vi "N-Channel N-Samples (2D DBL).vi"() -> ()   [LabVIEW 2019]
uses:
  <vilib>/DAQmx/read.llb/DAQmx Read (Analog 2D DBL NChan NSamp).vi
  <vilib>/DAQmx/create/channels.llb/DAQmx Create Channel (AI-Voltage-Basic).vi
  <vilib>/DAQmx/configure/timing.llb/DAQmx Timing (Sample Clock).vi
  <vilib>/DAQmx/miscellaneous.llb/DAQmx Fill In Error Info.vi
  <resource>/objmgr/daqmx.rc
panel:
  out "2D Array Indicator":dbl[][](array[numeric])
  out "Waveform Chart":dbl[][](graph)=[[2.0496230964079714, 1.4590899380474258, 1.1688589129306926], [1.792809839167455, 1.6428113650929288, 1.063875240333262], [1.977294228949858, 1.4178899502548294, 1.2041077913754692], [1.772057252723777, 1.6145817438276315, 1.1557359538560137], [1.804254280220954, 1.4838099307229835, 1.2335581530198065], [1.9325846125675221, 1.425977355265969, 0.957060457167272], [1.8865016632587663, 1.5289773247474594, 1.2024292733542894], [2.006744590594195, 1.5054780724509416, 1.108890041810358], [2.000793481246376, 1.3791314432203132, 0.9949034089175085], [1.7641224402600177, 1.5585802789391765, 1.010773033845027], [1.9341105380413222, 1.6245002594073306, 1.0701315347758416], [1.8980986968596454, 1.5283669545579395, 0.9697256385998108], [1.8352305673390912, 1.3620410779137546, 1.1365092928861353], [1.987670522171697, 1.4418469801934874, 1.0683004242072818], [1.9989623706778161, 1.5900143436994538, 0.934324167607654], [1.8655964842677084, 1.4720603045747245, 1.0792870876186407], [1.9122898037659841, 1.4857936338389233, 1.1467329935605945], [1.7418439283425398, 1.3936277352214117, 1.1227759636219368], [1.814020203253273, 1.4423047578356274, 1.1482589190343944], [1.8874172185430464, 1.4397106845301675, 1.1658070619830927], [1.8831446272164067, 1.3383892330698568, 1.08600115970336], [1.8190557573168127, 1.368144779808954, 1.0686056093020417], [1.9718008972441785, 1.424298837244789, 1.0715048677022614], [1.9710379345072786, 1.598406933805353, 0.9096041749320963], [1.7139194921720022, 1.4496292001098667, 0.9318826868495743], [1.9399090548417615, 1.5921506393627736, 1.0080263679921873], [1.7699209570604573, 1.381420331431013, 0.9009063997314372], [1.8753624073000275, 1.4758751182592242, 0.9627063814203314], [1.8892483291116062, 1.5924558244575335, 1.1323892941068758], [1.9069490646076845, 1.4687032685323649, 1.0504470961638233], [1.8732261116367077, 1.2892544328135014, 0.9527878658406324], [1.8730735190893277, 1.5356913968321788, 1.0397656178472243], [1.902829065828425, 1.5253151036103396, 0.945158238471633], [1.8997772148808252, 1.3528855250709555, 0.8984649189733573], [1.9202246162297434, 1.3434247871333964, 1.0531937620166631], [1.695913571581164, 1.5047151097140417, 1.1447492904446548], [1.9379253517258217, 1.4616840113528855, 0.8897671437726982], [1.8291268654438917, 1.4529862361522263, 1.1578722495193334], [1.9544053468428602, 1.381878109073153, 1.0357982116153448], [1.8515579699087497, 1.4844203009125034, 1.0507522812585832], [1.6920987578966644, 1.509292886135441, 1.0930204168828395], [1.9147312845240638, 1.2579729606006043, 0.9648426770836512], [1.705374309518723, 1.3516647846919156, 1.1029389324625385], [1.7534409619434186, 1.52302621539964, 1.096987823114719], [1.84789574877163, 1.2689596240119632, 0.9541611987670522], [1.7032380138554033, 1.2480544450209052, 1.0696737571337016], [1.7998290963469343, 1.3875240333262124, 0.9515671254615925], [1.8552201910458692, 1.4752647480697043, 0.9192175054170354], [1.8445387127292703, 1.5352336191900389, 0.9071626941740165], [1.7909787285988952, 1.2878810998870815, 0.968047120578631], [1.8315683462019714, 1.4183477278969696, 0.9179967650379955], [1.8291268654438917, 1.3315225684377574, 0.9793389690847499], [1.8506424146244698, 1.4864040040284432, 0.9111301004058961], [1.8674275948362682, 1.358073671681875, 1.0202337717825862], [1.7647328104495377, 1.2656025879696036, 1.044648579363384], [1.6786706137272256, 1.4389477217932676, 0.8099612414929654], [1.695150608844264, 1.4079714346751304, 0.9442426831873532], [1.7459639271217993, 1.426129947813349, 0.8490249336222419], [1.903134250923185, 1.4503921628467666, 1.0206915494247262], [1.728263191625721, 1.2985625782036805, 0.9382915738395337], [1.6559343241676077, 1.337626270332957, 0.8296456801049836], [1.6965239417706839, 1.3119907223731193, 1.0574663533433026], [1.6003906369212928, 1.4745017853328044, 0.8018738364818262], [1.7770928067873164, 1.4621417889950254, 0.9065523239844966], [1.760917996765038, 1.4735862300485245, 1.073946348460341], [1.8454542680135502, 1.249580370494705, 1.0556352427747429], [1.8408764915921507, 1.1912900173955503, 0.9602649006622517], [1.6621906186101871, 1.2094485305337688, 0.9547715689565721], [1.8057802056947538, 1.337015900143437, 0.8429212317270425], [1.7589342936490981, 1.2982573931089205, 0.9389019440290536], [1.6678365428632465, 1.4319284646137882, 0.7687612537003693], [1.717429120761742, 1.3324381237220375, 0.97872859889523], [1.7383342997528, 1.4278084658345287, 0.7548753318887905], [1.7766350291451765, 1.207464827417829, 0.8069093905453658], [1.6893520920438245, 1.401715140232551, 0.8729819635608996], [1.7703787347025972, 1.4052247688222907, 1.031983397930845], [1.6158024842066714, 1.3667714468825343, 0.9190649128696554], [1.8079165013580736, 1.2868129520554217, 0.9646900845362713], [1.6374706259346294, 1.314279610583819, 0.7527390362254708], [1.6692098757896665, 1.1691640980254525, 0.8868678853724784], [1.6875209814752647, 1.261787774285104, 0.9971922971282082], [1.5604113895077365, 1.3863032929471724, 0.8954130680257576], [1.6109195226905118, 1.1764885402996919, 0.8285775322733238], [1.6774498733481857, 1.4075136570329905, 0.8178960539567247], [1.8033387249366741, 1.1914426099429303, 0.8165227210303049], [1.8124942777794733, 1.2384411145359662, 0.7480086672566911], [1.7775505844294566, 1.1926633503219704, 0.913724173711356], [1.5301980651264993, 1.3428144169438765, 0.825830866420484], [1.6054261909848322, 1.3451033051545762, 0.8124027222510453], [1.6991180150761436, 1.3650929288613545, 0.826288644062624], [1.7670216986602374, 1.3003936887722403, 0.9662160100100711], [1.5895565660573137, 1.131168553727836, 0.7670827356791894], [1.6031373027741325, 1.3098544267097996, 0.8284249397259438], [1.5240943632312998, 1.2036500137333292, 0.7240516373180333], [1.7290261543626209, 1.1070589312417982, 0.9436323129978332], [1.5916928617206336, 1.3824884792626728, 0.7036042359691153], [1.7848750267036957, 1.346629230628376, 0.7521286660359509], [1.563921018097476, 1.1549729911191138, 0.7942442091128269], [1.7876216925565356, 1.3399151585436568, 0.9152500991851558], [1.6267891476180303, 1.08600115970336, 0.9396649067659536], [1.771446882534257, 1.1441389202551346, 0.9147923215430158], [1.5825373088778345, 1.3055818353831599, 0.6946012756736961], [1.5686513870662557, 1.1772515030365918, 0.9314249092074343], [1.73970763267922, 1.1685537278359326, 0.7600634784997101], [1.5619373149815363, 1.292764061403241, 0.9329508346812342], [1.717581713309122, 1.128269295327616, 0.6982634968108158], [1.6278572954496902, 1.2744529557176427, 0.9063997314371166], [1.4951017792291024, 1.2630085146641439, 0.7371745963927122], [1.4766380809961241, 1.1674855800042725, 0.9208960234382153], [1.6582232123783074, 1.3133640552995391, 0.8124027222510453], [1.5594958342234566, 1.152378917813654, 0.9169286172063357], [1.5952024903103732, 1.1154515213476974, 0.7209997863704337], [1.5506454664754172, 1.163060396130253, 0.749687185277871], [1.4766380809961241, 1.2344737083040864, 0.6935331278420362], [1.7117831965086825, 1.0626544999542222, 0.6682027649769585], [1.6933194982757043, 1.1105685598315378, 0.7773064363536485], [1.6782128360850856, 1.1680959501937926, 0.684377574999237], [1.6319772942289499, 1.3016144291512803, 0.8011108737449263], [1.4885402996917632, 1.19602038636433, 0.6324961088900418], [1.5906247138889738, 1.0403759880367442, 0.7918027283547472], [1.5659047212134158, 1.1232337412640767, 0.8751182592242195], [1.609698782311472, 1.3037507248146, 0.880458998382519], [1.4645832697531052, 1.1482589190343944, 0.6122013000885037], [1.4598529007843257, 1.1975463118381298, 0.6041138950773645], [1.4923551133762627, 1.250648518326365, 0.6295968504898221], [1.6133610034485917, 1.2971892452772606, 0.7138279366435744], [1.6928617206335643, 1.2111270485549486, 0.6306649983214819], [1.6844691305276651, 1.0197759941404463, 0.8867152928250984], [1.4323862422559281, 1.19647816400647, 0.6486709189123203], [1.674245429853206, 1.237830744346446, 0.7324442274239327], [1.63167210913419, 1.2022766808069094, 0.804620502334666], [1.555070650349437, 1.163212988677633, 0.6375316629535813], [1.6452528458510087, 1.077150791955321, 0.7486190374462112], [1.3948484756004518, 1.1152989288003174, 0.8285775322733238], [1.5710928678243354, 1.1009552293465987, 0.6002990813928648], [1.6130558183538315, 1.2340159306619465, 0.7968382824182867], [1.6823328348643452, 1.2707907345805232, 0.7515182958464308], [1.5901669362468338, 1.0889004181035797, 0.6591998046815394], [1.3846247749259926, 1.0037537766655475, 0.7267983031708731], [1.3823358867152928, 1.1554307687612537, 0.5595568712424085], [1.5150914029358806, 1.2424085207678457, 0.6707968382824183], [1.444898831141087, 0.9802545243690298, 0.6814783165990173], [1.5852839747306742, 1.0681478316599018, 0.5703909421063875], [1.4801477095858637, 1.098666341135899, 0.6944486831263161], [1.4398632770775475, 1.1455122531815547, 0.6692709128086184], [1.4505447553941466, 1.0248115482039857, 0.6099124118778039], [1.6159550767540514, 1.0567033906064027, 0.7219153416547136], [1.5465254676961577, 1.0557878353221228, 0.7379375591296121], [1.4592425305948058, 1.0895107882930997, 0.8192693868831447], [1.5381328775902585, 1.1360515152439954, 0.5378887295144505], [1.5478988006225776, 1.0504470961638233, 0.8011108737449263], [1.4841151158177435, 0.9833063753166296, 0.7771538438062685], [1.5939817499313333, 1.2140263069551682, 0.5423139133884701], [1.3719595934934539, 1.1838129825739312, 0.5117954039124729], [1.5205847346415602, 1.1449018829920348, 0.630512405774102], [1.349070711386456, 1.0928678243354595, 0.6881923886837367], [1.4313180944242683, 1.0611285744804224, 0.7553331095309305], [1.5225684377575, 1.043427838984344, 0.500198370311594], [1.4973906674398023, 1.0951567125461592, 0.6622516556291391], [1.381878109073153, 1.119113742484817, 0.6460768456068605], [1.5578173162022766, 1.0846278267769403, 0.5041657765434736], [1.3794366283150732, 1.1143833735160376, 0.7475508896145512], [1.3655507065034944, 1.0255745109408856, 0.7116916409802545], [1.4217047639393292, 1.1421552171391949, 0.5710013122959074], [1.5846736045411542, 1.1893063142796105, 0.7097079378643147], [1.5250099185155797, 1.1647389141514328, 0.5536057618945891], [1.5613269447920164, 1.1700796533097324, 0.6990264595477157], [1.4914395580919828, 0.9918515579699088, 0.5252235480819116], [1.3156529435102389, 0.9384441663869136, 0.5066072573015534], [1.3306070131534775, 0.9042634357737968, 0.5694753868221076], [1.545152134769738, 1.1581774346140934, 0.6540116580706198], [1.2970366527298807, 1.1140781884212776, 0.630054628131962], [1.5623950926236763, 1.1221655934324168, 0.6021301919614246], [1.293374431592761, 1.0362559892574847, 0.6495864741966002], [1.4065981017487106, 1.012451551866207, 0.685750907925657], [1.3306070131534775, 1.0245063631092257, 0.7147434919278542], [1.5582750938444165, 1.1256752220221564, 0.6324961088900418], [1.477553636280404, 0.9967345194860683, 0.4518265327921384], [1.5268410290841394, 1.0731833857234412, 0.5714590899380474], [1.5166173284096804, 0.9300515762810144, 0.6648457289345988], [1.476943266090884, 1.0890530106509597, 0.44724875637073885], [1.3771477401043732, 1.1278115176854762, 0.5259865108188116], [1.3773003326517532, 0.9155552842799157, 0.5667287209692679], [1.294595171971801, 0.8458204901272622, 0.48509170812097535], [1.30481887264626, 0.8986175115207373, 0.6961272011474959], [1.2649922177800836, 0.9936826685384685, 0.5796990874965666], [1.381572923978393, 1.076235236671041, 0.6897183141575366], [1.2765892513809625, 0.9843745231482894, 0.4426709799493393], [1.2753685110019226, 1.1014130069887387, 0.6497390667439802], [1.3441877498702963, 0.9897152623065889, 0.46571245460371713], [1.4200262459181494, 1.0521256141850033, 0.6849879451887569], [1.3704336680196538, 1.0472426526688436, 0.6064027832880642], [1.41285439619129, 1.0818811609241004, 0.631275368511002], [1.466872157963805, 1.0469374675740837, 0.576647236548967], [1.403698843348491, 0.9912411877803888, 0.6170842616046632], [1.5111239967040009, 0.9952085940122685, 0.44709616382335887], [1.4937284463026825, 1.0930204168828395, 0.38529618213446454], [1.336710715048677, 0.8883938108462782, 0.5926694540238655], [1.3969847712637715, 0.8359019745475631, 0.3985717337565233], [1.3884395886104923, 0.9266945402386547, 0.5159154026917325], [1.3753166295358135, 1.0812707907345804, 0.4664754173406171], [1.260414441358684, 1.0364085818048647, 0.4686117130039369], [1.317178868984039, 1.0400708029419843, 0.6051820429090243], [1.41315958128605, 0.8420056764427626, 0.564287240211188], [1.1970885341959898, 0.7966856898709067, 0.37003692739646593], [1.2634662923062838, 0.9276100955229346, 0.5041657765434736], [1.2866603595080417, 1.0203863643299662, 0.48295541245765555], [1.3121433149204993, 0.9207434308908353, 0.6234931485946227], [1.4056825464644307, 1.0289315469832454, 0.4881435590685751], [1.337168492690817, 0.8362071596423231, 0.4858546708578753], [1.1700796533097324, 0.9607226783043916, 0.5957213049714651], [1.292306283761101, 0.9918515579699088, 0.6070131534775841], [1.2088381603442488, 0.858790856654561, 0.41657765434736166], [1.2298959318826868, 0.9595019379253518, 0.4425183874019593], [1.2706381420331432, 1.0350352488784447, 0.6231879634998627], [1.2651448103274636, 1.0234382152775658, 0.45365764336069825], [1.4096499526963102, 0.967284157841731, 0.39063692129276406], [1.3518173772392956, 0.7689138462477493, 0.6031983397930845], [1.2158574175237282, 0.9617908261360515, 0.3553880428479873], [1.2709433271279031, 1.0112308114871669, 0.575579088717307], [1.2259285256508072, 0.9912411877803888, 0.4791405987731559], [1.4050721762749108, 0.9804071169164098, 0.402233954893643], [1.4101077303384502, 0.8595538193914609, 0.39216284676656393], [1.2952055421613209, 0.8928189947202979, 0.42649616992706074], [1.3455610827967162, 0.9686574907681509, 0.4142887661366619], [1.3084810937833795, 0.7454145939512314, 0.41596728415784173], [1.3824884792626728, 0.9152500991851558, 0.3979613635670034], [1.2166203802606281, 0.9669789727469711, 0.3573717459639271], [1.3234351634266182, 0.8606219672231208, 0.38453321939756463], [1.3280129398480178, 0.8169804986724448, 0.4770043031098361], [1.208227790154729, 0.8346812341685232, 0.41596728415784173], [1.1767937253944518, 0.7452620014038515, 0.3741569261757256], [1.1713003936887723, 0.6944486831263161, 0.2708517715994751], [1.184881130405591, 0.7940916165654469, 0.554826502273629], [1.2298959318826868, 0.7867671742912076, 0.3944517349772637], [1.313974425489059, 0.9143345439008759, 0.36255989257484666], [1.2445448164311654, 0.7155064546647542, 0.3514206366161077], [1.349375896481216, 0.8970915860469375, 0.34180730613116855], [1.1606189153721733, 0.9112826929532761, 0.42847987304300056], [1.1500900296029541, 0.9372234260078738, 0.49684133426923427], [1.2787255470442824, 0.7902768028809473, 0.3563035981322672], [1.1934263130588703, 0.8766441846980193, 0.5380413220618305], [1.292916653950621, 0.8027893917661062, 0.47029023102511675], [1.1720633564256722, 0.8717612231818598, 0.3979613635670034], [1.0794396801660207, 0.8507034516434218, 0.4971465193639943], [1.1116367076631977, 0.8107242042298655, 0.2739036225470748], [1.1935789056062502, 0.836817529831843, 0.511490218817713], [1.1981566820276497, 0.8339182714316232, 0.25513473921933655], [1.317178868984039, 0.7197790459913938, 0.45152134769737845], [1.1799981688894314, 0.8919034394360179, 0.260628070925016], [1.3135166478469191, 0.7560960722678305, 0.2897732474745933], [1.0701315347758416, 0.684377574999237, 0.37888729514450514], [1.2320322275460067, 0.8098086489455855, 0.23133030182805872], [1.066774498733482, 0.7571642200994904, 0.4112369151890622], [1.0885952330088198, 0.6787316507461776, 0.42344431897946105], [1.2611774040955839, 0.8665730765709403, 0.2996917630542924]]
  out "Waveform Graph":dbl[][](graph)
  out "Actual Sample Rate (Hz)":dbl
  in  "Desired Sample Rate (Hz)":dbl=2560.0
  in  "Number of Samples":i32=256
  in  "Stop":bool
  in  "Physical Channels":tag="PCI-6221/ai0, PCI-6221/ai2:3"
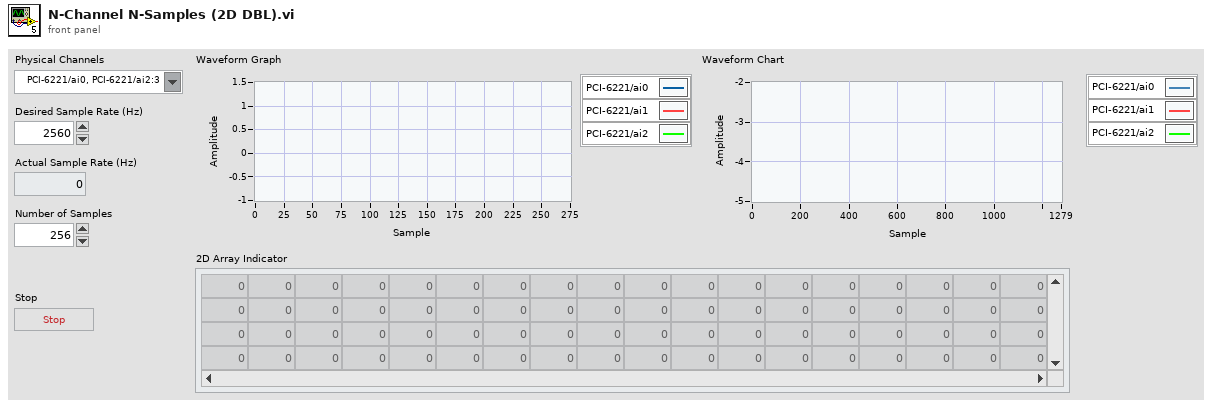
[diagram p1: front panel]
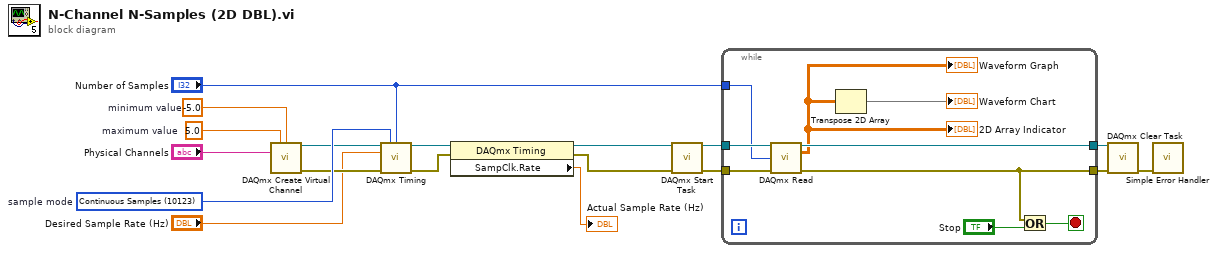
[diagram p0: block diagram]
diagram:
  w13 = 5.0  # maximum value
  w14 = -5.0  # minimum value
  w18 = 10123 items=["Finite Samples"=10178, "Continuous Samples"=10123, "Hardware Timed Single Point"=12522]  # sample mode
  n1 = call-poly <vilib>:"DAQmx Create Virtual Channel.vi"("maximum value"=w13, "minimum value"=w14, "physical channels"="Physical Channels") -> ("task out"=w17:refnum<k21>, "error out"=w16:errorcluster)  [unwired: 11 in]
  n2 = call-poly <vilib>:"DAQmx Timing.vi"("task/channels in"=w17, "sample mode"=w18, "samples per channel"="Number of Samples", "rate"="Desired Sample Rate (Hz)", "error in"=w16) -> ("task out"=w5:refnum<k21>, "error out"=w4:errorcluster)  [unwired: 9 in]
  n3 = property class="DAQmx Timing"(reference=w5, error in=w4) -> (reference out=w3:refnum<k21>, error out=w2:errorcluster, "SampClk.Rate"=→"Actual Sample Rate (Hz)":dbl)
  n4 = call <vilib>:"DAQmx Start Task.vi"("task/channels in"=w3, "error in"=w2) -> ("task out"=w9:refnum<k21>, "error out"=w8:errorcluster)  [unwired: 12 in]
  n5 = while {
    tunnel: [w27] -> w12
    tunnel: [w26] -> w11
    tunnel: w9 -> [w23]
    tunnel: w8 -> [w22]
    tunnel: "Number of Samples" -> [w21]
    stop <- w24 stop-if-true
    n6 = call-poly <vilib>:"DAQmx Read.vi"("task/channels in"=w23, "number of samples per channel"=w21, "error in"=w22) -> ("task out"=w27:refnum<k21>, "data"=w19:dbl[][], "error out"=w26:errorcluster)  [unwired: 10 in]
    "Waveform Graph" <- w19
    "2D Array Indicator" <- w19
    n7 = Transpose 2D Array(2D array=w19) -> (transposed array=→"Waveform Chart":dbl[][])
    n8 = Or(x=w26, y="Stop") -> (x .or. y?=w24:bool)
  }
  n9 = call <vilib>:"DAQmx Clear Task.vi"("task in"=w12, "error in"=w11) -> ("error out"=w10:errorcluster)  [unwired: 13 in]
  n10 = call <vilib>:"Simple Error Handler.vi"("error in (no error)"=w10) -> ()  [unwired: 4 in, 5 out]
